vi "PXI Configuration.vi"(3 "names":T1) -> (0 "Master Clock":tag="/PXI1Slot2/ai/SampleClock", 1 "Tasks Configuration":T2[](array[typedef]))   [LabVIEW 2013]
uses:
  Telemanipulation/PXI/Task Definition.ctl
  Telemanipulation/PXI/Task Types.ctl
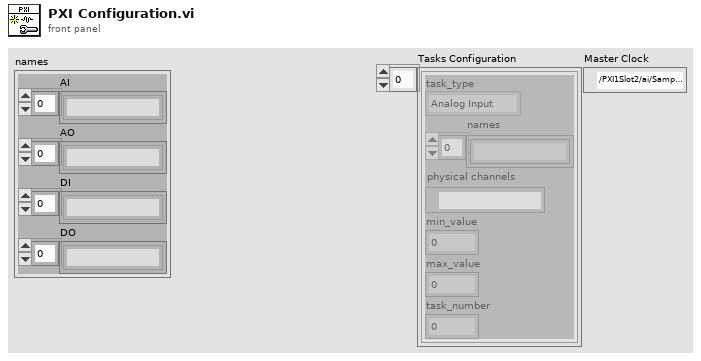
[diagram p1: front panel]
types:
  T1 = cluster{"AI":string[], "AO":string[], "DI":string[], "DO":string[]}
  T2 = typedef "Task Definition.ctl" = cluster{"task_type":T3, "names":string[], "physical channels":tag, "min_value":dbl, "max_value":dbl, "task_number":i32}
  T3 = typedef "Task Types.ctl" = enum16{"Analog Input", "Analog Output", "Digital Input", "Digital Output"}
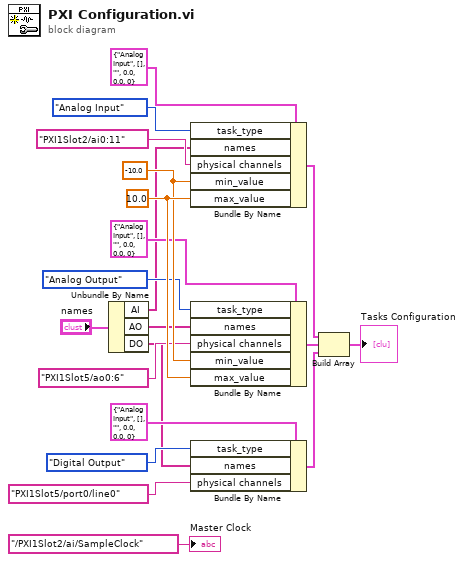
[diagram p0: block diagram]
diagram:
  w15 = -10.0 ("min_value")
  w16 = 10.0 ("max_value")
  n1 = Unbundle By Name("names") -> ("AI"=w1:string[], "AO"=w2:string[], "DO"=w3:string[])
  n2 = Bundle By Name(cluster=T2 {"task_type"=enum."Analog Input", "names"=[], "physical channels"="", "min_value"=0.0, "max_value"=0.0, "task_number"=0} ("task_definition"), "task_type"=Task_Types."Analog Input", "names"=w1, "physical channels"=tag "PXI1Slot2/ai0:11", "min_value"=w15, "max_value"=w16) -> (w7:T2)
  n3 = Bundle By Name(cluster=T2 {"task_type"=enum."Analog Input", "names"=[], "physical channels"="", "min_value"=0.0, "max_value"=0.0, "task_number"=0} ("task_definition"), "task_type"=Task_Types."Analog Output", "names"=w2, "physical channels"=tag "PXI1Slot5/ao0:6", "min_value"=w15, "max_value"=w16) -> (w10:T2)
  n4 = Bundle By Name(cluster=T2 {"task_type"=enum."Analog Input", "names"=[], "physical channels"="", "min_value"=0.0, "max_value"=0.0, "task_number"=0} ("task_definition"), "task_type"=Task_Types."Digital Output", "names"=w3, "physical channels"=tag "PXI1Slot5/port0/line0") -> (w19:T2)
  n5 = Build Array(w7, w10, w19) -> (→"Tasks Configuration":T2[])
  "Master Clock" <- tag "/PXI1Slot2/ai/SampleClock" ("Master Clock")
